vi "MC Mode Set and Channel commands.vi"() -> ()   [LabVIEW 2009]
uses:
  <vilib>/Instr/_visa.llb/VISA Configure Serial Port (Instr).vi
panel:
  out "Heartbeat":bool
  out "All Stop":bool
  out "Set Mode 3":bool
  in  "Mode command 3":string="^04 C0"
  out "Set Mode 2":bool
  in  "Mode command 2":string="^03 00"
  in  "Mode command 1":string="^01 C4"
  out "Set RS232 Control":bool
  out "Set Mode 1":bool
  in  "Stop":bool
  in  "Channel A cmd":i32(slide)=1 min=-127 max=127 step=1 scale=-127.0..127.0
  in  "Channel B cmd":i32(slide)=1 min=-127 max=127 step=1 scale=-127.0..127.0
  in  "VISA resource name":refnum<visa-resource-name>="COM3"
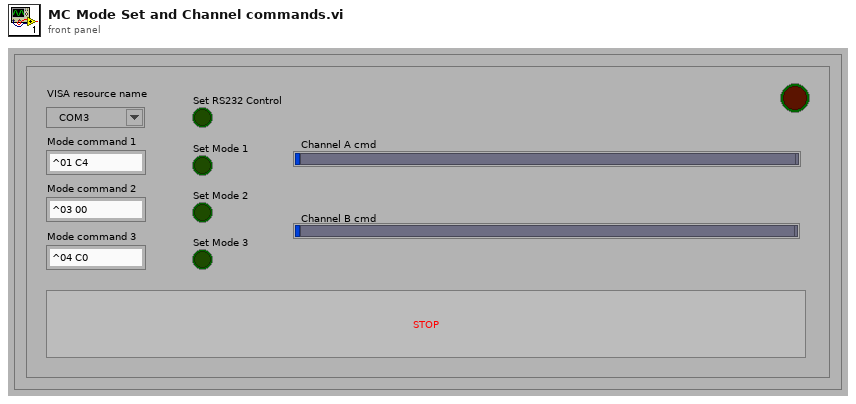
[diagram p1: front panel]
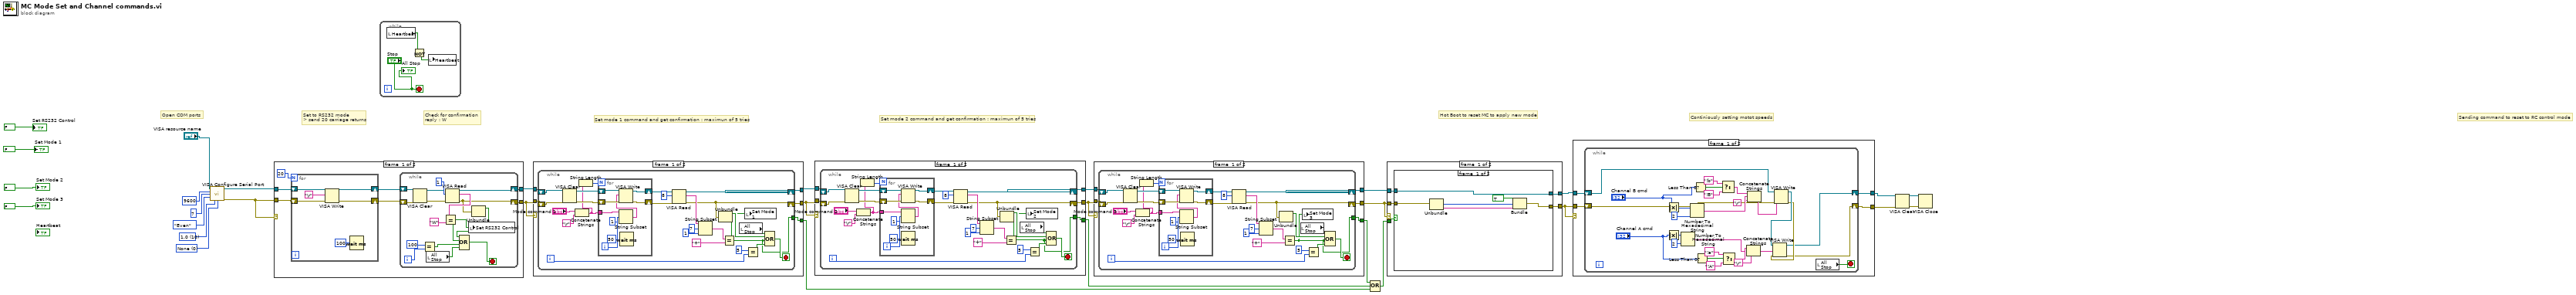
[diagram p0: block diagram]
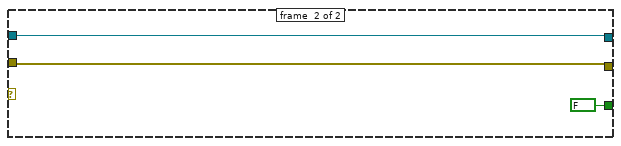
[diagram p2: hidden frame]
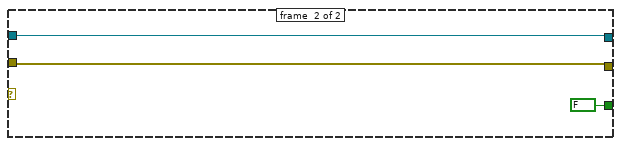
[diagram p3: hidden frame]
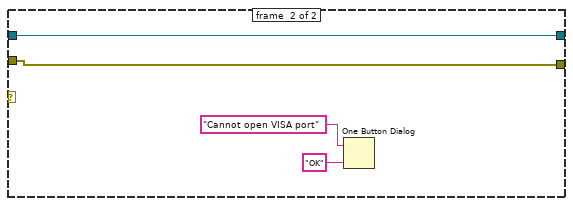
[diagram p5: hidden frame]
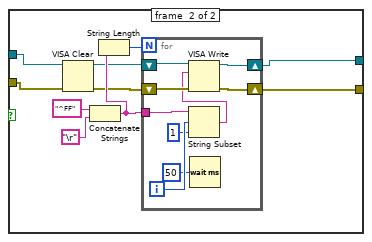
[diagram p6: hidden frame]
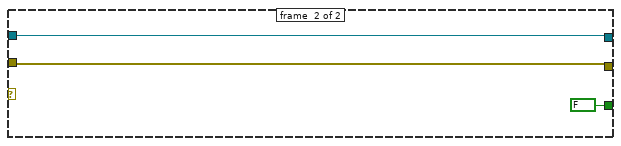
[diagram p8: hidden frame]
diagram:
  w25 = u16 0 items=["None", "XON/XOFF", "RTS/CTS", "XON/XOFF & RTS/CTS", "DTR/DSR", "XON/XOFF & DTR/DSR"] ("flow control (0:none)")
  w26 = u16 10 items=["1.0"=10, "1.5"=15, "2.0"=20] ("stop bits (10: 1 bit)")
  # "Continiously setting motot speeds"
  # "Sending command to reset to RC control mode"
  # "Set mode 2 command and get confirmation : maximun of 5 tries"
  # "Hot Boot to reset MC to apply new mode"
  # "Check for confirmation\nreply : W"
  # "Set mode 1 command and get confirmation : maximun of 5 tries"
  # "Set to RS232 mode\n> send 20 carriage returns"
  # "Open COM ports"
  n1 = call-poly "VISA Configure Serial Port"("VISA resource name"="VISA resource name", "baud rate (9600)"=u32 9600, "data bits (8)"=u16 7, "parity (0:none)"=enum16{"None", "Odd", "Even", "Mark", "Space"}."Even", "stop bits (10: 1 bit)"=w26, "flow control (0:none)"=w25) -> ("VISA resource name out"=w24:refnum<visa-resource-name>, "error out"=w20:errorcluster)  [unwired: 1 in, 7 out]
  n2 = case shown="No Error" w20 {
    tunnel: w20 -> [w36 w62]
    tunnel: w24 -> [w35 w63]
    tunnel: [w34 w63] -> w23
    tunnel: [w31 w62] -> w21
    frame #0 {
      n3 = for {
        N: 20 -> [_]
        shift-right: [w56] -> w33
        shift-left: w36 -> [w59]
        shift-right: [w58] -> w32
        shift-left: w35 -> [w57]
        n4 = VISA Write(VISA resource name=w57, write buffer="\r", error in (no error)=w59) -> (VISA resource name out=w58:refnum<visa-resource-name>, error out=w56:errorcluster)  [unwired: 1 out]
        n5 = Wait (ms)(milliseconds to wait=u32 100) -> ()  [unwired: 1 out]
      }
      n6 = while {
        shift-right: [w49] -> w34
        shift-left: w32 -> [w50]
        shift-right: [w41] -> w31
        shift-left: w33 -> [w48]
        i -> [w45]
        stop <- w42 stop-if-true
        n7 = VISA Clear(VISA resource name=w50, error in (no error)=w48) -> (VISA resource name out=w47:refnum<visa-resource-name>, error out=w40:errorcluster)
        n8 = Equal?(x=100, y=w45) -> (x = y?=w43:bool)
        n9 = local read "All Stop"() -> (w38:bool)
        n10 = VISA Read(VISA resource name=w47, byte count=u32 1, error in (no error)=w40) -> (VISA resource name out=w49:refnum<visa-resource-name>, read buffer=w52:string, error out=w41:errorcluster)  [unwired: 1 out]
        n11 = Equal?(x=w52, y="W") -> (x = y?=w39:bool)
        n12 = local write "Set RS232 Control"(w39) -> ()
        n13 = Unbundle(w41) -> ("status"=w46:bool)  [unwired: 2 out]
        n14 = Compound Arithmetic op=OR(w46, w39, w43, w38) -> (w42:bool)
      }
    }
    frame #1 {
      n15 = One Button Dialog(message="Cannot open VISA port", button name ("OK")="OK") -> ()  [unwired: 1 out]
    }
  }
  n16 = while {
    stop <- "Stop" stop-if-true
    n17 = local read "Heartbeat"() -> (w65:bool)
    n18 = Not(x=w65) -> (.not. x?=w64:bool)
    n19 = local write "Heartbeat"(w64) -> ()
    "All Stop" <- "Stop"
  }
  n20 = case shown="No Error" w21 {
    tunnel: [w71 w108] -> w13
    tunnel: [w70 w107] -> w14
    tunnel: w23 -> [w69 w108]
    tunnel: w21 -> [w68 w107]
    tunnel: [w67 FALSE] -> w15
    frame #0 {
      n21 = while {
        shift-right: [w92] -> w71
        shift-left: w69 -> [w96]
        shift-right: [w79] -> w70
        shift-left: w68 -> [w95]
        tunnel: [w73] -> w67
        i -> [w76]
        stop <- w74 stop-if-true
        n22 = VISA Clear(VISA resource name=w96, error in (no error)=w95) -> (VISA resource name out=w89:refnum<visa-resource-name>, error out=w88:errorcluster)
        n23 = Concatenate Strings("Mode command 1", "\r") -> (w80:string)
        n24 = String Length(string=w80) -> (length=w81:i32)
        n25 = for {
          N: w81 -> [_]
          tunnel: w80 -> [w101]
          shift-right: [w105] -> w94
          shift-left: w88 -> [w102]
          shift-right: [w104] -> w93
          shift-left: w89 -> [w103]
          i -> [w100]
          n26 = String Subset(string=w101, offset (0)=w100, length (rest)=1 ("length (rest)")) -> (substring=w98:string)
          n27 = VISA Write(VISA resource name=w103, write buffer=w98, error in (no error)=w102) -> (VISA resource name out=w104:refnum<visa-resource-name>, error out=w105:errorcluster)  [unwired: 1 out]
          n28 = Wait (ms)(milliseconds to wait=u32 50) -> ()  [unwired: 1 out]
        }
        n29 = VISA Read(VISA resource name=w93, byte count=u32 8, error in (no error)=w94) -> (VISA resource name out=w92:refnum<visa-resource-name>, read buffer=w85:string, error out=w79:errorcluster)  [unwired: 1 out]
        n30 = String Subset(string=w85, offset (0)=7, length (rest)=1 ("length (rest)")) -> (substring=w84:string)
        n31 = Unbundle(w79) -> ("status"=w75:bool)  [unwired: 2 out]
        n32 = Equal?(x=w84, y="+") -> (x = y?=w73:bool)
        n33 = local read "All Stop"() -> (w72:bool)
        n34 = local write "Set Mode 1"(w73) -> ()
        n35 = Equal?(x=5, y=w76) -> (x = y?=w77:bool)
        n36 = Compound Arithmetic op=OR(w72, w75, w73, w77) -> (w74:bool)
      }
    }
    frame #1 {
    }
  }
  n37 = case shown="No Error" w14 {
    tunnel: [w113 w150] -> w10
    tunnel: [w112 w149] -> w9
    tunnel: w13 -> [w111 w150]
    tunnel: w14 -> [w110 w149]
    tunnel: [w109 FALSE] -> w11
    frame #0 {
      n38 = while {
        shift-right: [w134] -> w113
        shift-left: w111 -> [w138]
        shift-right: [w121] -> w112
        shift-left: w110 -> [w137]
        tunnel: [w115] -> w109
        i -> [w118]
        stop <- w116 stop-if-true
        n39 = VISA Clear(VISA resource name=w138, error in (no error)=w137) -> (VISA resource name out=w131:refnum<visa-resource-name>, error out=w130:errorcluster)
        n40 = Concatenate Strings("Mode command 2", "\r") -> (w122:string)
        n41 = String Length(string=w122) -> (length=w123:i32)
        n42 = for {
          N: w123 -> [_]
          tunnel: w122 -> [w143]
          shift-right: [w147] -> w136
          shift-left: w130 -> [w144]
          shift-right: [w146] -> w135
          shift-left: w131 -> [w145]
          i -> [w142]
          n43 = String Subset(string=w143, offset (0)=w142, length (rest)=1 ("length (rest)")) -> (substring=w140:string)
          n44 = VISA Write(VISA resource name=w145, write buffer=w140, error in (no error)=w144) -> (VISA resource name out=w146:refnum<visa-resource-name>, error out=w147:errorcluster)  [unwired: 1 out]
          n45 = Wait (ms)(milliseconds to wait=u32 50) -> ()  [unwired: 1 out]
        }
        n46 = VISA Read(VISA resource name=w135, byte count=u32 8, error in (no error)=w136) -> (VISA resource name out=w134:refnum<visa-resource-name>, read buffer=w127:string, error out=w121:errorcluster)  [unwired: 1 out]
        n47 = String Subset(string=w127, offset (0)=7, length (rest)=1 ("length (rest)")) -> (substring=w126:string)
        n48 = Unbundle(w121) -> ("status"=w117:bool)  [unwired: 2 out]
        n49 = Equal?(x=w126, y="+") -> (x = y?=w115:bool)
        n50 = local read "All Stop"() -> (w114:bool)
        n51 = local write "Set Mode 2"(w115) -> ()
        n52 = Equal?(x=5, y=w118) -> (x = y?=w119:bool)
        n53 = Compound Arithmetic op=OR(w114, w117, w115, w119) -> (w116:bool)
      }
    }
    frame #1 {
    }
  }
  n54 = case shown="No Error" w9 {
    tunnel: [w155 w192] -> w7
    tunnel: [w154 w191] -> w3
    tunnel: w10 -> [w153 w192]
    tunnel: w9 -> [w152 w191]
    tunnel: [w151 FALSE] -> w6
    frame #0 {
      n55 = while {
        shift-right: [w176] -> w155
        shift-left: w153 -> [w180]
        shift-right: [w163] -> w154
        shift-left: w152 -> [w179]
        tunnel: [w157] -> w151
        i -> [w160]
        stop <- w158 stop-if-true
        n56 = VISA Clear(VISA resource name=w180, error in (no error)=w179) -> (VISA resource name out=w173:refnum<visa-resource-name>, error out=w172:errorcluster)
        n57 = Concatenate Strings("Mode command 3", "\r") -> (w164:string)
        n58 = String Length(string=w164) -> (length=w165:i32)
        n59 = for {
          N: w165 -> [_]
          tunnel: w164 -> [w185]
          shift-right: [w189] -> w178
          shift-left: w172 -> [w186]
          shift-right: [w188] -> w177
          shift-left: w173 -> [w187]
          i -> [w184]
          n60 = String Subset(string=w185, offset (0)=w184, length (rest)=1 ("length (rest)")) -> (substring=w182:string)
          n61 = VISA Write(VISA resource name=w187, write buffer=w182, error in (no error)=w186) -> (VISA resource name out=w188:refnum<visa-resource-name>, error out=w189:errorcluster)  [unwired: 1 out]
          n62 = Wait (ms)(milliseconds to wait=u32 50) -> ()  [unwired: 1 out]
        }
        n63 = VISA Read(VISA resource name=w177, byte count=u32 8, error in (no error)=w178) -> (VISA resource name out=w176:refnum<visa-resource-name>, read buffer=w169:string, error out=w163:errorcluster)  [unwired: 1 out]
        n64 = String Subset(string=w169, offset (0)=7, length (rest)=1 ("length (rest)")) -> (substring=w168:string)
        n65 = Unbundle(w163) -> ("status"=w159:bool)  [unwired: 2 out]
        n66 = Equal?(x=w168, y="+") -> (x = y?=w157:bool)
        n67 = local read "All Stop"() -> (w156:bool)
        n68 = local write "Set Mode 3"(w157) -> ()
        n69 = Equal?(x=5, y=w160) -> (x = y?=w161:bool)
        n70 = Compound Arithmetic op=OR(w156, w159, w157, w161) -> (w158:bool)
      }
    }
    frame #1 {
    }
  }
  n71 = Compound Arithmetic op=OR(w6, w11, w15) -> (w16:bool)
  n72 = case shown="No Error" w3 {
    tunnel: w3 -> [w197 w224]
    tunnel: w7 -> [w196 w223]
    tunnel: w16 -> [w193 _]
    tunnel: [w195 w224] -> w19
    tunnel: [w194 w223] -> w30
    frame #0 {
      n73 = case shown="True" w193 {
        tunnel: w197 -> [w202 w207]
        tunnel: w196 -> [w198 w206]
        tunnel: [w203 w205] -> w195
        tunnel: [w198 w204] -> w194
        frame #0 {
          n74 = Unbundle(w202) -> ("code"=w200:i32, "source"=w201:string)  [unwired: 1 out]
          n75 = Bundle(TRUE, "code"=w200, "source"=w201) -> (w203:cluster{bool, "code":i32, "source":string})  [unwired: 1 out]
        }
        frame #1 {
          n76 = VISA Clear(VISA resource name=w206, error in (no error)=w207) -> (VISA resource name out=w210:refnum<visa-resource-name>, error out=w211:errorcluster)
          n77 = Concatenate Strings("^FF" ("string"), "\r") -> (w213:string)
          n78 = String Length(string=w213) -> (length=w212:i32)
          n79 = for {
            N: w212 -> [_]
            tunnel: w213 -> [w218]
            shift-right: [w222] -> w205
            shift-left: w211 -> [w219]
            shift-right: [w221] -> w204
            shift-left: w210 -> [w220]
            i -> [w217]
            n80 = String Subset(string=w218, offset (0)=w217, length (rest)=1 ("length (rest)")) -> (substring=w215:string)
            n81 = VISA Write(VISA resource name=w220, write buffer=w215, error in (no error)=w219) -> (VISA resource name out=w221:refnum<visa-resource-name>, error out=w222:errorcluster)  [unwired: 1 out]
            n82 = Wait (ms)(milliseconds to wait=u32 50) -> ()  [unwired: 1 out]
          }
        }
      }
    }
    frame #1 {
    }
  }
  n83 = case shown="No Error" w19 {
    tunnel: w19 -> [w228 w256]
    tunnel: [w227 w257] -> w2
    tunnel: [w226 w256] -> w1
    tunnel: w30 -> [w225 w257]
    frame #0 {
      n84 = while {
        shift-right: [w233] -> w227
        shift-left: w225 -> [w238]
        shift-right: [w232] -> w226
        shift-left: w228 -> [w237]
        stop <- w229 stop-if-true
        n85 = Absolute Value(x="Channel B cmd") -> (abs(x)=w255:i32)
        n86 = Absolute Value(x="Channel A cmd") -> (abs(x)=w254:i32)
        n87 = Number To Hexadecimal String(1:i16 2 ("width (-)"), 2:w254) -> (0:w240:string)
        n88 = Number To Hexadecimal String(1:i16 2 ("width (-)"), 2:w255) -> (0:w242:string)
        n89 = Less Than 0?(x="Channel B cmd") -> (x < 0?=w251:bool)
        n90 = Less Than 0?(x="Channel A cmd") -> (x < 0?=w245:bool)
        n91 = Select(t="!b", s=w251, f="!B") -> (s? t:f=w243:string)
        n92 = Select(t="!a", s=w245, f="!A") -> (s? t:f=w241:string)
        n93 = Concatenate Strings(w241, w240, "\r") -> (w236:string)
        n94 = Concatenate Strings(w243, w242, "\r") -> (w239:string)
        n95 = VISA Write(VISA resource name=w238, write buffer=w239, error in (no error)=w237) -> (VISA resource name out=w235:refnum<visa-resource-name>, error out=w234:errorcluster)  [unwired: 1 out]
        n96 = VISA Write(VISA resource name=w235, write buffer=w236, error in (no error)=w234) -> (VISA resource name out=w233:refnum<visa-resource-name>, error out=w232:errorcluster)  [unwired: 1 out]
        n97 = local read "All Stop"() -> (w229:bool)
      }
    }
    frame #1 {
    }
  }
  n98 = VISA Clear(VISA resource name=w2, error in (no error)=w1) -> (VISA resource name out=w5:refnum<visa-resource-name>, error out=w4:errorcluster)
  n99 = VISA Close(VISA resource name=w5, error in (no error)=w4) -> ()  [unwired: 1 out]
  "Set Mode 1" <- FALSE
  "Set RS232 Control" <- FALSE
  "Set Mode 2" <- FALSE
  "Set Mode 3" <- FALSE
